vi "sub_vi_get_linear_parameters.vi"(8 "error in":errorcluster, 11 "VISA resource name in":refnum<visa-resource-name>) -> (0 "error out":errorcluster, 1 "intercept_2":dbl, 2 "slope_2":dbl, 3 "VISA resource name out":refnum<visa-resource-name>, 4 "intercept_1":dbl, 5 "slope_1":dbl, 6 "intercept_0":dbl, 7 "slope_0":dbl)   [LabVIEW 2019]
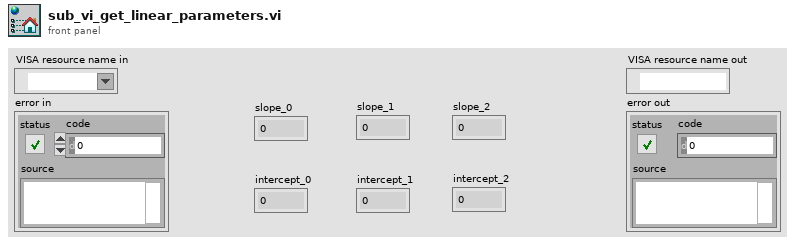
[diagram p1: front panel]
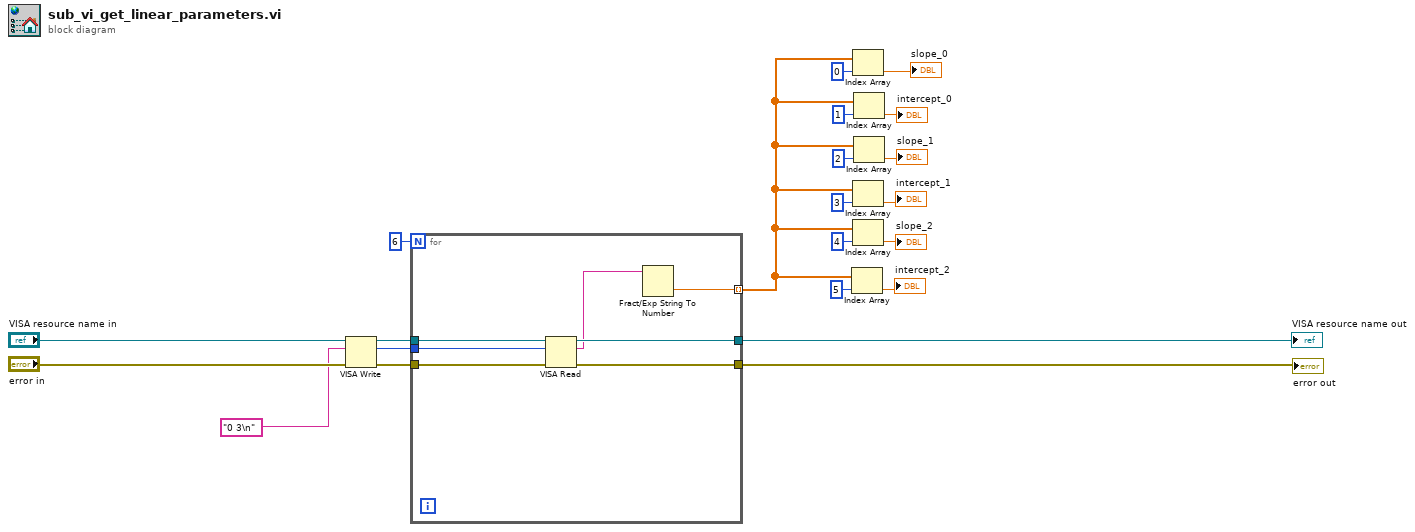
[diagram p0: block diagram]
diagram:
  n1 = VISA Write(VISA resource name="VISA resource name in", write buffer="0 3\n", error in (no error)="error in") -> (VISA resource name out=w16:refnum<visa-resource-name>, return count=w17:u32, error out=w18:errorcluster)
  n2 = for {
    N: 6 -> [_]
    tunnel: w18 -> [w29]
    tunnel: w17 -> [w28]
    tunnel: w16 -> [w27]
    tunnel: [w26] -> w20
    tunnel: [w25] -> w19
    tunnel: [w23] -> w3 mode=indexing
    n3 = VISA Read(VISA resource name=w27, byte count=w28, error in (no error)=w29) -> (VISA resource name out=w26:refnum<visa-resource-name>, read buffer=w24:string, error out=w25:errorcluster)  [unwired: 1 out]
    n4 = Fract/Exp String To Number(string=w24) -> (number=w23:dbl)  [unwired: 3 in, 1 out]
  }
  "VISA resource name out" <- w20
  "error out" <- w19
  n5 = Index Array(array=w3, index=5) -> (element=→"intercept_2":dbl)
  n6 = Index Array(array=w3, index=0) -> (element=→"slope_0":dbl)
  n7 = Index Array(array=w3, index=3) -> (element=→"intercept_1":dbl)
  n8 = Index Array(array=w3, index=4) -> (element=→"slope_2":dbl)
  n9 = Index Array(array=w3, index=1) -> (element=→"intercept_0":dbl)
  n10 = Index Array(array=w3, index=2) -> (element=→"slope_1":dbl)
